vi "deinitialize.vi"(0 "HGF_Rendezvous":refnum<class "HGF_Rendezvous.lvclass">, 5 "error in (no error)":errorcluster) -> (19 "error out":errorcluster)   [LabVIEW 2014, in "HGF_BaseClasses.lvlib" / "HGF_Rendezvous.lvclass"]
doc: "This is a dynamic dispatch VI. It can be overwritten by childclasses to release allocated recources."
uses:
  HGF_Rendezvous.lvclass
  HGF_InternalEvent/HGF_InternalEvent.lvclass
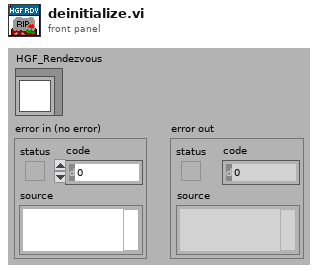
[diagram p1: front panel]
types:
  T1 = typedef "Rendezvous RefNum" = refnum<k1>
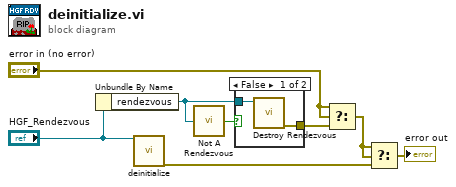
[diagram p0: block diagram]
diagram:
  n1 = Unbundle By Name("HGF_Rendezvous") -> ("rendezvous"=w2:T1)
  n2 = call-parent "deinitialize.vi"("HGF_Factory"="HGF_Rendezvous") -> ("error out"=w5:errorcluster)  [unwired: 1 in, 17 out]
  n3 = call <vilib>:"Not A Rendezvous.vi"("rendezvous"=w2) -> ("not a rendezvous"=w1:bool)
  n4 = case shown="False" w1 {
    tunnel: w2 -> [w10 _]
    tunnel: [w9 _] -> w6
    frame False {
      n5 = call <vilib>:"Destroy Rendezvous.vi"("rendezvous"=w10) -> ("error out"=w9:errorcluster)  [unwired: 1 in, 5 out]
    }
    frame True {
    }
  }
  n6 = Select(t="error in (no error)", s="error in (no error)", f=w6) -> (s? t:f=w4:errorcluster)
  n7 = Select(t=w4, s=w4, f=w5) -> (s? t:f=→"error out":errorcluster)
